vi "Day 6 Puzzle 1.vi"(11 "Path":path) -> ()   [LabVIEW 2021]
uses:
  <vilib>/Utility/file.llb/Read Delimited Spreadsheet (string).vi
panel:
  out "Array 4":bool[](array[boolean])
  out "Array 3":bool[](array[boolean])
  out "Array 2":string[](array[string])
  out "String":string
  out "Array":string[](array[string])
  out "Numeric":i32
  out "element":string
  out "all rows":string[][](array[string])
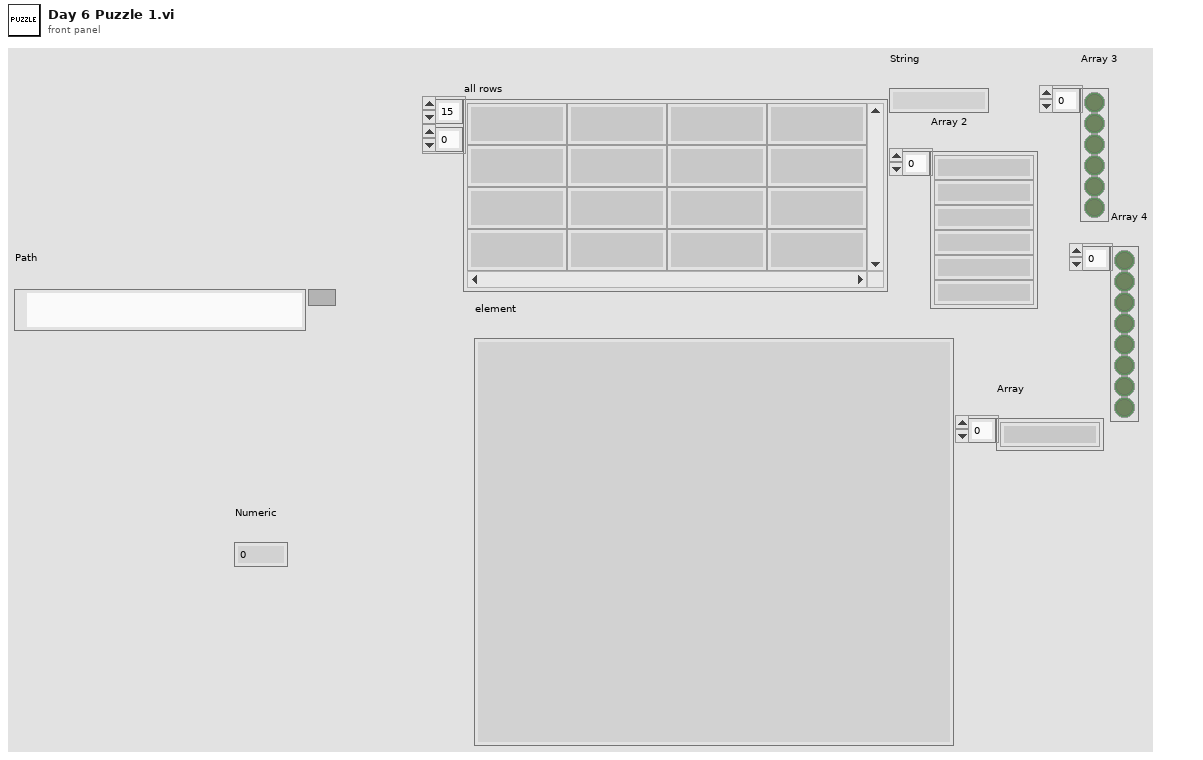
[diagram p1: front panel]
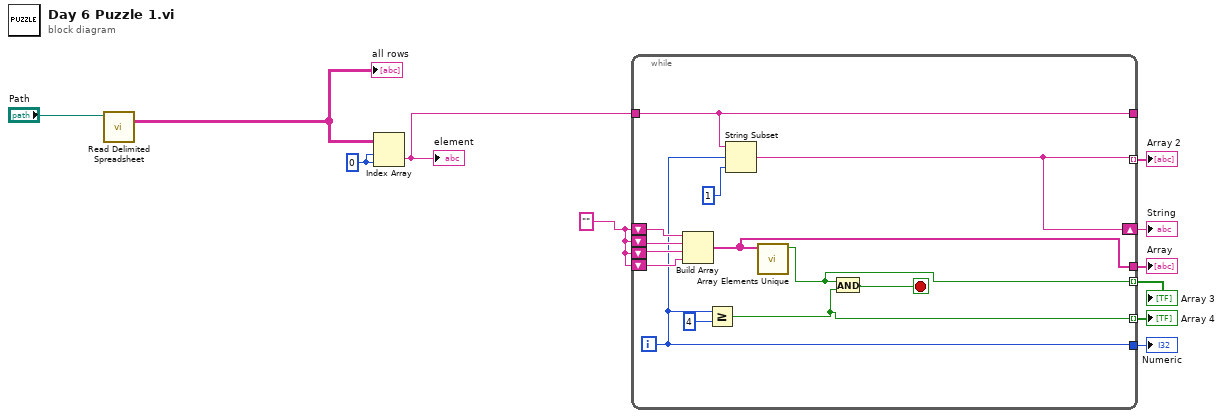
[diagram p0: block diagram]
diagram:
  w7 = "" ("String")
  w9 = 0 ("disabled index (col)")
  n1 = call-poly <vilib>:"Read Delimited Spreadsheet.vi"("file path (dialog if empty)"="Path") -> ("all rows"=w10:string[][])  [unwired: 9 in, 5 out]
  "all rows" <- w10
  n2 = Index Array(array=w10, index (row)=w9, index (col)=w9) -> (element=w8:string)
  "element" <- w8
  n3 = while {
    shift-right: [w14] -> w4
    shift-left: w7 -> [w23]
    shift-left: w7 -> [w20]
    shift-left: w7 -> [w21]
    shift-left: w7 -> [w22]
    tunnel: [w16] -> w6
    tunnel: [w17] -> w5
    tunnel: w8 -> [w19]
    tunnel: [w19] -> _
    tunnel: [w14] -> w3 mode=indexing
    tunnel: [w13] -> w2 mode=indexing
    tunnel: [w12] -> w1 mode=indexing
    i -> [w16]
    stop <- w15 stop-if-true
    n4 = Build Array(w23, w22, w21, w20) -> (w17:string[])
    n5 = Greater Or Equal?(x=w16, y=4) -> (x >= y?=w12:bool)
    n6 = String Subset(string=w19, offset (0)=w16, length (rest)=1 ("length (rest)")) -> (substring=w14:string)
    n7 = call "Array Elements Unique"("Array"=w17) -> ("result"=w13:bool)  [unwired: 10 in]
    n8 = And(x=w13, y=w12) -> (x .and. y?=w15:bool)
  }
  "Numeric" <- w6
  "Array" <- w5
  "String" <- w4
  "Array 2" <- w3
  "Array 3" <- w2
  "Array 4" <- w1
